vi "FdxCmdEDESubDestroyCvi.vi"(8 "error in":errorcluster, 9 "EDESubsciriberHandle":u32, 11 "InstrumentHandle":u32) -> (0 "error out":errorcluster, 3 "InstrumentHandle":u32)   [LabVIEW 2020, in "AIM664LV.lvlib"]
doc: "This function is used to remove and release all resources associated with an EDE Subscriber."
uses:
  AIM664LV.lvlib
  AFDX_LibraryAdmin/FdxGlobalDllPath.vi
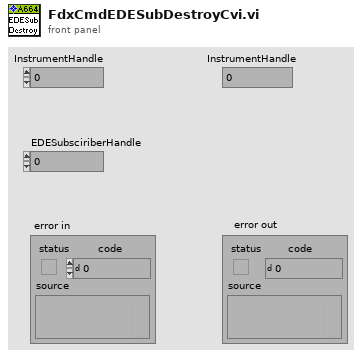
[diagram p1: front panel]
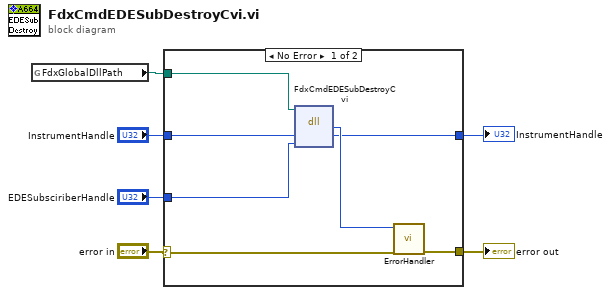
[diagram p0: block diagram]
diagram:
  n1 = global read "FdxGlobalDllPath.vi" "FdxGlobalDllPath"() -> (w4:path)
  n2 = case shown="No Error" "error in" {
    selector: "error in" -> [w12 w15]
    tunnel: [w13 w15] -> w6
    tunnel: w4 -> [w10 _]
    tunnel: "InstrumentHandle" -> [w9 w14]
    tunnel: [w8 w14] -> w2
    tunnel: "EDESubsciriberHandle" -> [w7 _]
    frame No Error {
      n3 = dll-call lib="aim_fdx.19.dll" fn="FdxCmdEDESubDestroyCvi"(path in=w10, "InstrumentHandle"=w9, "EDESubscriberHandle"=w7) -> ("status"=w11:i32, "InstrumentHandle"=w8:u32)  [unwired: 3 in, 2 out]
      n4 = call "ErrorHandler.vi"("error in"=w12, "AIM Error"=w11) -> ("error out"=w13:errorcluster)  [unwired: 9 in]
    }
    frame Error {
    }
  }
  "error out" <- w6
  "InstrumentHandle" <- w2
